vi "SSL Detection Balls Invalidate.vi"(11 "Value":T1[](array[typedef])) -> (3 "Array":T1[](array[typedef]))   [LabVIEW 2018]
uses:
  Controls/SSL Detection Ball.ctl
  <vilib>/Analysis/Matrix/Datatypes/RealMatrix.ctl
  <vilib>/Analysis/Matrix/NI_Matrix.lvlib
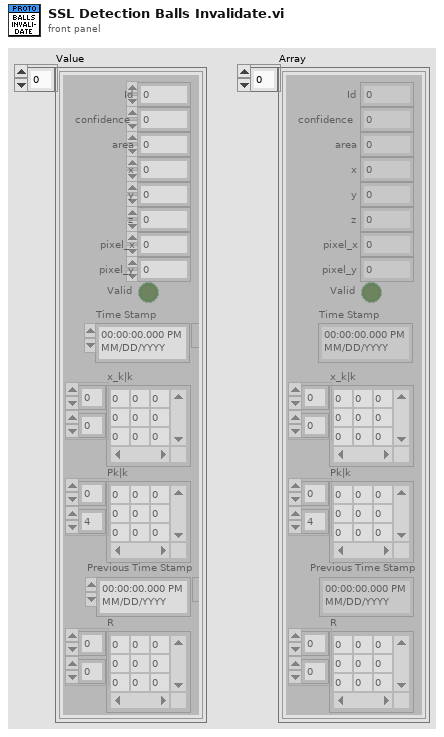
[diagram p1: front panel]
types:
  T1 = typedef "SSL Detection Ball.ctl" = cluster{"x":sgl, "area":u32, "confidence":sgl, "y":sgl, "z":sgl, "pixel_x":sgl, "pixel_y":sgl, "Valid":bool, "Time Stamp":timestamp, "x_k|k":T2, "Pk|k":T2, "Id":u32, "Previous Time Stamp":timestamp, "R":T2}
  T2 = typedef "NI_Matrix.lvlib/RealMatrix.ctl" = dbl[][]
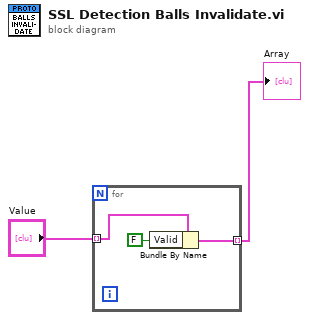
[diagram p0: block diagram]
diagram:
  n1 = for {
    tunnel: "Value" -> [w5] mode=indexing
    tunnel: [w3] -> w2 mode=indexing
    n2 = Bundle By Name(cluster=w5, "Valid"=FALSE) -> (w3:T1)
  }
  "Array" <- w2
